vi "更新t2.vi"(8 "error in (no error)":errorcluster caption="错误输入（无错误）") -> (0 "error out":errorcluster caption="错误输出")   [LabVIEW 2014]
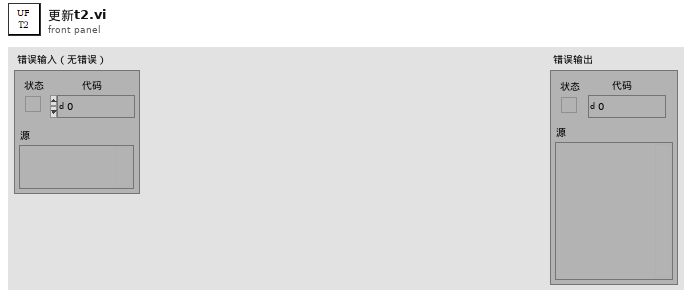
[diagram p1: front panel]
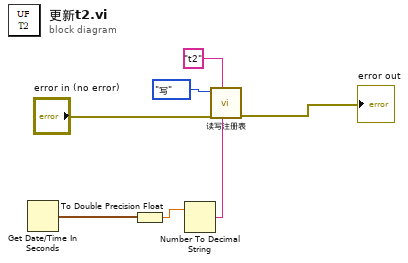
[diagram p0: block diagram]
diagram:
  n1 = Get Date/Time In Seconds() -> (seconds since 1Jan1904=w5:timestamp)
  n2 = To Double Precision Float(number=w5) -> (double precision float=w2:dbl)
  n3 = Number To Decimal String(number=w2) -> (decimal integer string=w1:string)  [unwired: 1 in]
  n4 = call "读写注册表.vi"("写入内容"=w1, "键名称"="t2", "error in (no error)"="error in (no error)", "读/写"=enum16{"读", "写"}."写") -> ("error out"=→"error out":errorcluster)  [unwired: 6 in, 1 out]
